vi "校验和.vi"(1 "输入（Hex）":string) -> (0 "输出":string)   [LabVIEW 2015, in "WZ5005E.lvlib"]
uses:
  WZ5005E.lvlib
panel:
  out "校验和":string
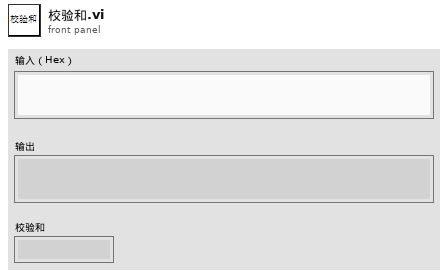
[diagram p1: front panel]
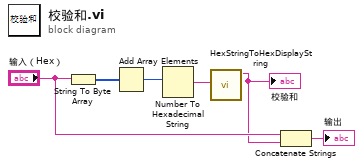
[diagram p0: block diagram]
diagram:
  n1 = String To Byte Array(string="输入（Hex）") -> (unsigned byte array=w6:u8[])
  n2 = Add Array Elements(numeric array=w6) -> (sum=w5:u8)
  n3 = Number To Hexadecimal String(2:w5) -> (0:w4:string)  [unwired: 1 in]
  n4 = call "HexStringToHexDisplayString.vi"("正常显示HEX字符串"=w4) -> ("HEX显示字符串"=w2:string)  [unwired: 10 in]
  "校验和" <- w2
  n5 = Concatenate Strings("输入（Hex）", w2) -> (→"输出":string)
